vi "RPM Needed.vi"(10 "Shooter Presets":T2 {"Shooter PID Gains"."D" format="%.3f"; "Shooter PID Gains"."I" format="%.3f"; "Shooter PID Gains"."P" format="%.3f"}, 11 "Shot Type":T1=enum."Dist Shot") -> (2 "RPM":dbl, 3 "Hood?":bool)   [LabVIEW 2016]
uses:
  Common Code/Shooter Presets.ctl
  Common Code/Shot Type.ctl
  Robot Global Data.vi
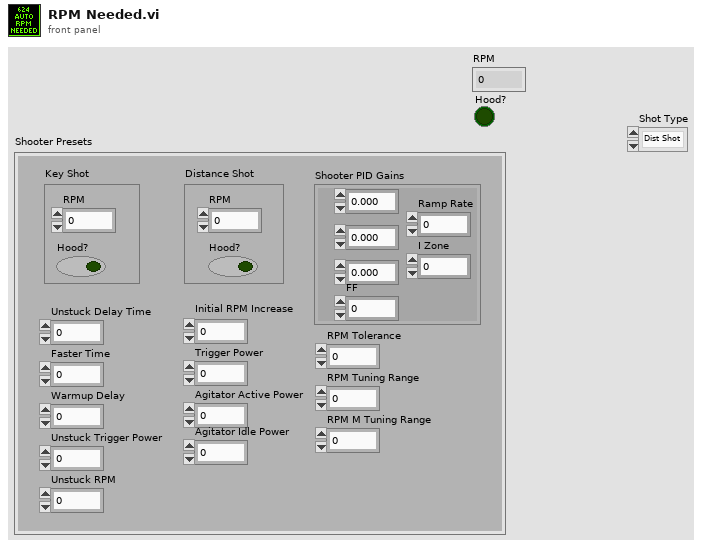
[diagram p1: front panel]
types:
  T1 = typedef "Shot Type.ctl" = enum16{"Vision Shot", "Dist Shot", "Key Shot"}
  T2 = typedef "Shooter Presets.ctl" = cluster{"Key Shot":cluster{"RPM ":dbl, "Hood?":bool}, "Distance Shot":cluster{"RPM":dbl, "Hood?":bool}, "RPM Tolerance":dbl, "Unstuck Delay Time ":dbl, "Initial RPM Increase":dbl, "Warmup Delay":dbl, "Faster Time":dbl, "Shooter PID Gains":cluster{"P":dbl, "I":dbl, "D":dbl, "FF":dbl, "Ramp Rate":dbl, "I Zone":dbl}, "Unstuck Trigger Power":dbl, "Trigger Power":dbl, "Unstuck RPM":dbl, "Agitator Active Power":dbl, "Agitator Idle Power":dbl, "RPM Tuning Range":dbl, "RPM M Tuning Range":dbl}
  T3 = typedef "Goal Vision Packet.ctl" = cluster{"Distance":dbl, "Angle":dbl, "Found Target?":bool}
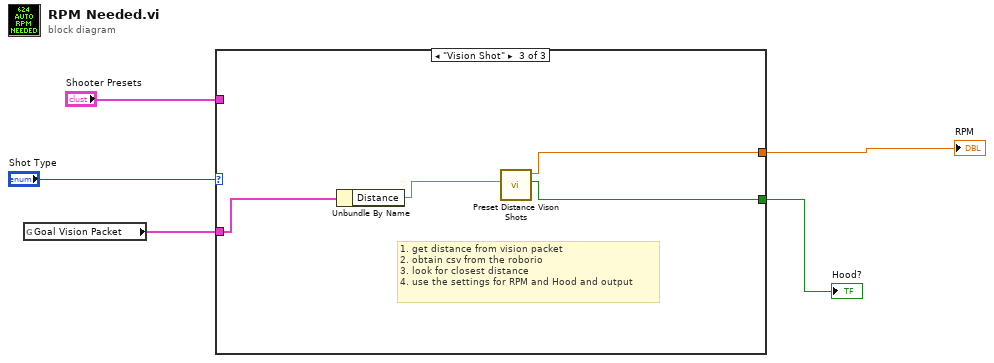
[diagram p0: block diagram]
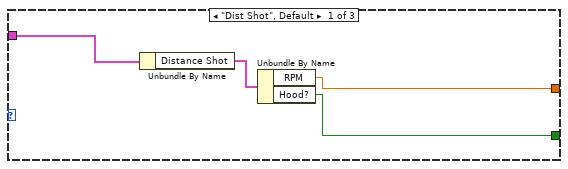
[diagram p2: hidden frame]
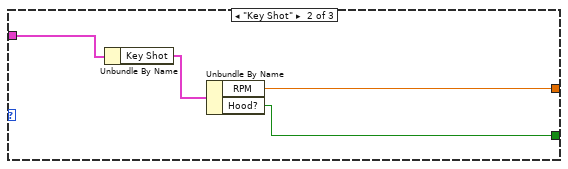
[diagram p3: hidden frame]
diagram:
  n1 = global read "Robot Global Data.vi" "Goal Vision Packet"() -> (w1:T3)
  n2 = case shown="\"Vision Shot\"" "Shot Type" {
    tunnel: "Shooter Presets" -> [w9 w13 _]
    tunnel: [w7 w11 w15] -> w3
    tunnel: [w6 w10 w14] -> w2
    tunnel: w1 -> [_ _ w17]
    frame "Dist Shot", Default {
      n3 = Unbundle By Name(w9) -> ("Distance Shot"=w8:cluster{"RPM":dbl, "Hood?":bool})
      n4 = Unbundle By Name(w8) -> ("RPM"=w7:dbl, "Hood?"=w6:bool)
    }
    frame "Key Shot" {
      n5 = Unbundle By Name(w13) -> ("Key Shot"=w12:cluster{"RPM ":dbl, "Hood?":bool})
      n6 = Unbundle By Name(w12) -> ("RPM"=w11:dbl, "Hood?"=w10:bool)
    }
    frame "Vision Shot" {
      # "1. get distance from vision packet\n2. obtain csv from the roborio\n3. look for closest distance\n4. use the settings for RPM and Hood and output"
      n7 = Unbundle By Name(w17) -> ("Distance"=w16:dbl)
      n8 = call "Preset Distance Vison Shots.vi"("Distance"=w16) -> ("Hood Down?"=w14:bool, "Shooter RPM"=w15:dbl)  [unwired: 9 in]
    }
  }
  "RPM" <- w3
  "Hood?" <- w2
